vi "Use Adaptive Filter (Point by Point).vi"() -> ()   [LabVIEW 2019]
doc: "This example demonstrates how to create and use an adaptive filter. This example simulates and filters signals in point-by-point mode.\n\nComplete the following steps to use this example.\n\n1. Run this VI. Observe how the coefficients of the adaptive filter converge to those of the unknown system.\n\n2. Browse the block diagram of this example to understand how this example uses the adaptive filter VIs.\n\n3. Replace the AFT Create FIR LMS VI with other filter creation VIs palette to try other adaptive filter algorithms.\n\nThis example uses an FIR LMS adaptive filter to identify the impulse response of an unknown system. A lowpass FIR filter simulates the unknown system. The input to both this system and the adaptive filter is Gaussian white noise. The output of this system is the reference of the adaptive filter."
uses:
  <vilib>/addons/Adaptive Filters/Create/AFT Create FIR LMS (Real).vi
  <vilib>/addons/Adaptive Filters/Processing/AFT Filter Signal and Update Coefficients (Real, PtByPt).vi
  <vilib>/addons/Adaptive Filters/Analysis/AFT Get Coefficients (FIR, Real).vi
  <vilib>/addons/Adaptive Filters/NI_AdaptiveFilter.lvlib
panel:
  out "Error Signal":dbl(graph)
  out "Coefficients":dbl[][](graph)
  in  "Stop":bool
  in  "Step Size":dbl=0.002 min=0.0 step=0.001
  in  "Filter Length":i32=25 min=2
  # "Select Help>>Show Context Help and move the cursor over the VI icon of this example for more information."
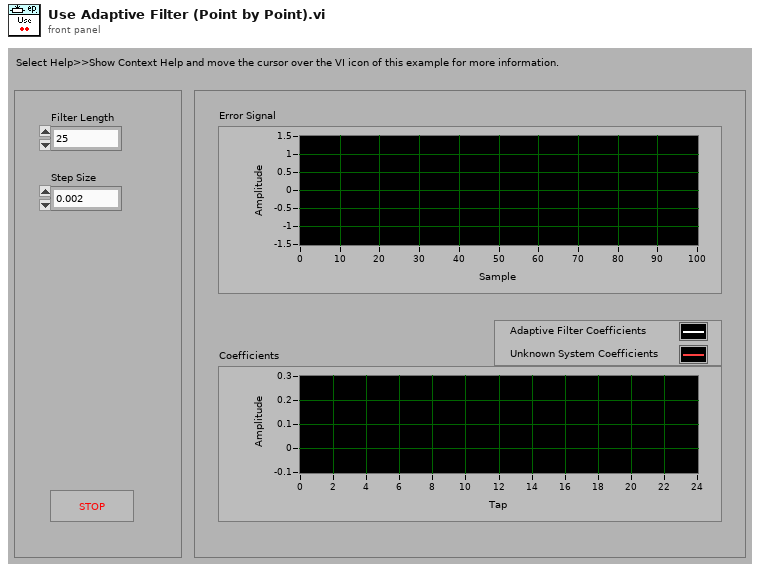
[diagram p1: front panel]
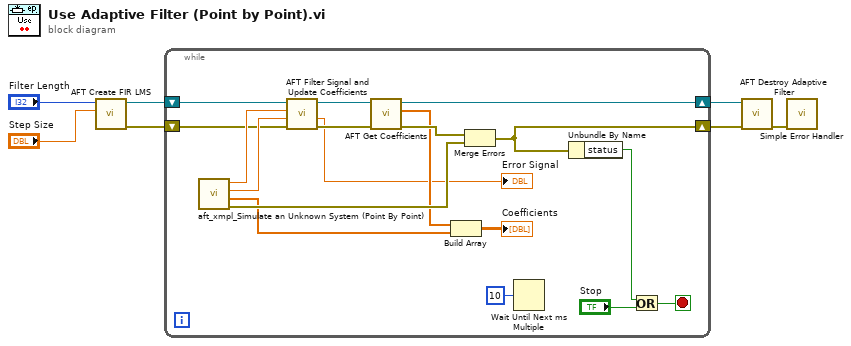
[diagram p0: block diagram]
diagram:
  n1 = call-poly <vilib>:"AFT Create FIR LMS.vi"("step size"="Step Size", "filter length"="Filter Length") -> ("error out"=w4:errorcluster, "adaptive filter out"=w5:refnum<k20>)  [unwired: 2 in, 6 out]
  n2 = while {
    shift-right: [w22] -> w3
    shift-left: w5 -> [w23]
    shift-right: [w10] -> w2
    shift-left: w4 -> [w11]
    stop <- w9 stop-if-true
    n3 = call "aft_xmpl_Simulate an Unknown System (Point By Point).vi"() -> ("error out"=w24:errorcluster, "unknown system coefficients"=w12:dbl[], "response signal"=w13:dbl, "stimulus signal"=w14:dbl)  [unwired: 1 in, 7 out]
    n4 = call-poly <vilib>:"AFT Filter Signal and Update Coefficients.vi"("error in (no error)"=w11, "d(n)"=w13, "x(n)"=w14, "adaptive filter in"=w23) -> ("error out"=w20:errorcluster, "e(n)"=→"Error Signal":dbl, "adaptive filter out"=w21:refnum<k20>)  [unwired: 2 in, 3 out]
    n5 = call-poly <vilib>:"AFT Get Coefficients.vi"("error in (no error)"=w20, "adaptive filter in"=w21) -> ("error out"=w25:errorcluster, "coefficients"=w19:dbl[], "adaptive filter out"=w22:refnum<k20>)  [unwired: 7 out]
    n6 = Build Array(w19, w12) -> (→"Coefficients":dbl[][])
    n7 = Merge Errors(w25, w24) -> (w10:errorcluster)
    n8 = Wait Until Next ms Multiple(millisecond multiple=u32 10) -> ()  [unwired: 1 out]
    n9 = Unbundle By Name(w10) -> ("status"=w8:bool)
    n10 = Or(x=w8, y="Stop") -> (x .or. y?=w9:bool)
  }
  n11 = call <vilib>:"AFT Destroy Adaptive Filter.vi"("error in (no error)"=w2, "adaptive filter in"=w3) -> ("error out"=w1:errorcluster)  [unwired: 9 out]
  n12 = call <vilib>:"Simple Error Handler.vi"("error in (no error)"=w1) -> ()  [unwired: 1 in, 8 out]
